vi "Compass.vi"(7 "GPS/Mag":bool, 8 "error in (no error)":errorcluster caption="Fehler (Eingang, kein Fehler)", 11 "SBG Data Cluster":T1) -> (0 "error out":errorcluster caption="Fehler (Ausgang)", 2 "Heading Digital":dbl format="%.1f", 3 "CompassGauge":picture)   [LabVIEW 2023]
uses:
  SBG Data Cluster.ctl
  <vilib>/Utility/miscctls.llb/LVBoundsTypeDef.ctl
  <vilib>/picture/picture.llb/imagedata.ctl
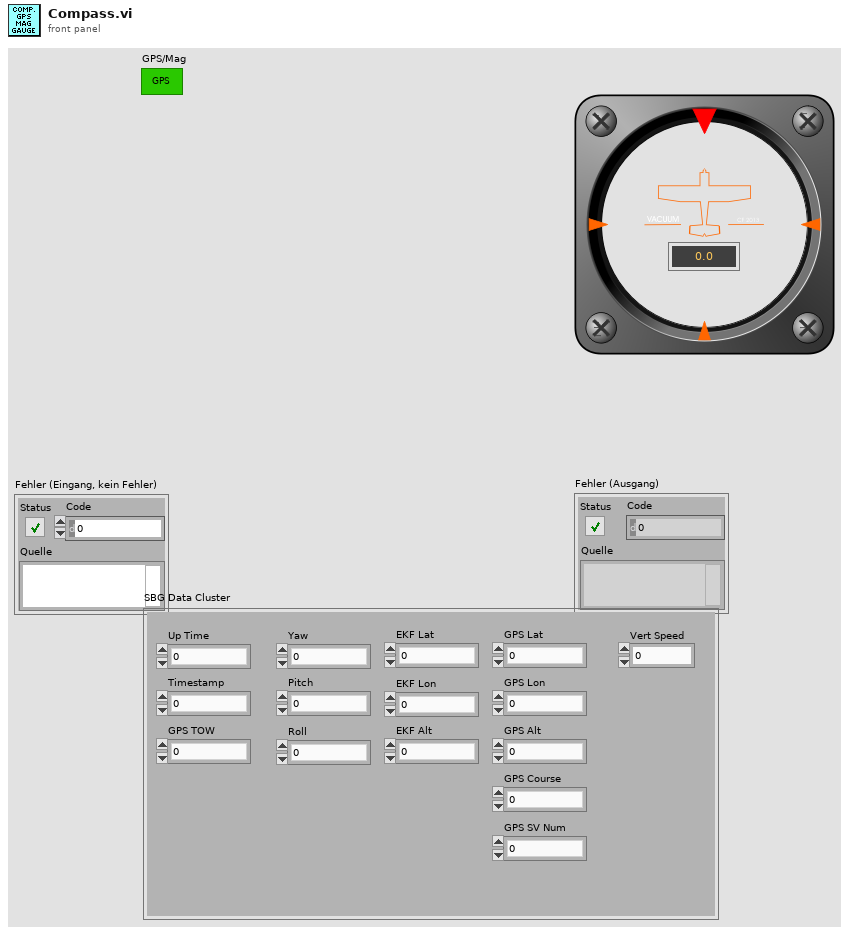
[diagram p1: front panel]
types:
  T1 = typedef "SBG Data Cluster.ctl" = cluster{"Up Time":u32, "Timestamp":u32, "Yaw":sgl, "Pitch":sgl, "Roll":sgl, "EKF Lat":dbl, "EKF Lon":dbl, "EKF Alt":dbl, "GPS Lat":dbl, "GPS Lon":dbl, "GPS Alt":dbl, "GPS Course":sgl, "GPS SV Num":u8, "GPS TOW":u32, "Vert Speed":dbl}
  T2 = typedef "LVBoundsTypeDef.ctl" = cluster{"Width":u32, "Height":u32}
  T3 = typedef "imagedata.ctl" = cluster{"image type":i32, "image depth":i32, "image":u8[], "mask":u8[], "colors":u32[], "Rectangle":cluster{"left":i16, "top":i16, "right":i16, "bottom":i16}}
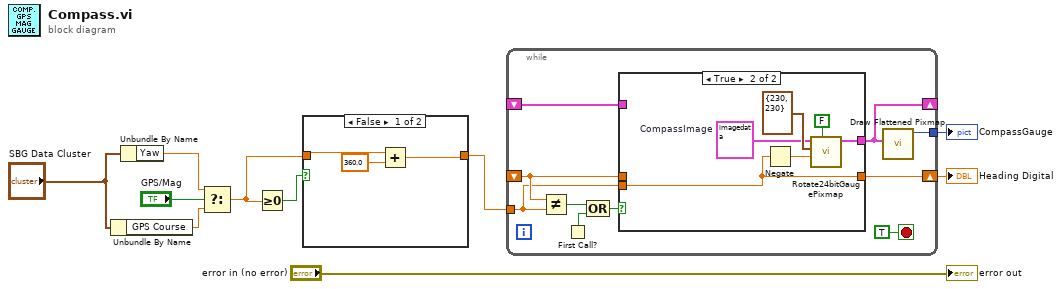
[diagram p0: block diagram]
diagram:
  n1 = Unbundle By Name("SBG Data Cluster") -> ("GPS Course"=w6:sgl)
  n2 = Unbundle By Name("SBG Data Cluster") -> ("Yaw"=w7:sgl)
  n3 = Select(t=w7, s="GPS/Mag", f=w6) -> (s? t:f=w1:sgl)
  n4 = Greater Or Equal To 0?(x=w1) -> (x >= 0?=w3:bool)
  n5 = case shown="False" w3 {
    tunnel: [w11 w14] -> w2
    tunnel: w1 -> [w13 w14]
    frame False {
      n6 = Add(x=w13, y=sgl 360.0) -> (x+y=w11:sgl)
    }
    frame True {
    }
  }
  n7 = while {
    shift-right: [w21] -> w9
    shift-left: _ -> [w20]
    tunnel: w2 -> [w15]
    shift-right: [w19] -> _
    shift-left: _ -> [w18]
    tunnel: [w16] -> w8
    stop <- TRUE stop-if-true
    n8 = Not Equal?(x=w20, y=w15) -> (x != y?=w22:bool)
    n9 = First Call?() -> (First Call?: T/F=w23:bool)
    n10 = Compound Arithmetic op=OR(w22, w23) -> (w24:bool)
    n11 = case shown="True" w24 {
      tunnel: [w26 w32] -> w19
      tunnel: w18 -> [w26 _]
      tunnel: w20 -> [w25 _]
      tunnel: [w25 w27] -> w21
      tunnel: w15 -> [_ w27]
      frame False {
      }
      frame True {
        w29 = T3 {"image type"=0, "image depth"=24, "image"=array[158700 elements], "mask"=[], "colors"=[], "Rectangle"={"left"=0, "top"=0, "right"=230, "bottom"=230}}  # CompassImage
        n12 = Negate(x=w27) -> (-x=w28:sgl)
        n13 = call "Rotate24bitGaugePixmap.vi"("Maske kombinieren? (F)"=FALSE, "Rotation Angle (degrees)"=w28, "Größe des Darstellungsbereichs"=T2 {"Width"=230, "Height"=230}, "image data"=w29) -> ("image data out"=w32:T3)  [unwired: 7 in]
      }
    }
    n14 = call <vilib>:"Draw Flattened Pixmap.vi"("image data"=w19) -> ("new picture"=w16:picture)  [unwired: 1 in, 7 out]
  }
  "Heading Digital" <- w9
  "CompassGauge" <- w8
  "error out" <- "error in (no error)"
